vi "LVClass_WavefrontCorrector Check and Move to Absolute Position.vi"(0 "WavefrontCorrector in":refnum<class "WavefrontCorrector.lvclass">, 5 "Position":T1, 7 "Sleep after command apply (ms)":i32, 9 "Mirror preferences.Wavefront Corrector State":T2[](array[typedef]), 11 "error in (no error)":errorcluster) -> (4 "WavefrontCorrector out":refnum<class "WavefrontCorrector.lvclass">, 15 "error out":errorcluster)   [LabVIEW 2020, in "WavefrontCorrector.lvclass"]
uses:
  WavefrontCorrector.lvclass
  Wavefront Corrector states - ONE.ctl
  Wavefront Corrector Position.ctl
  Wavefront Corrector states.ctl
  WavefrontCorrector.lvclass/WavefrontCorrector.ctl
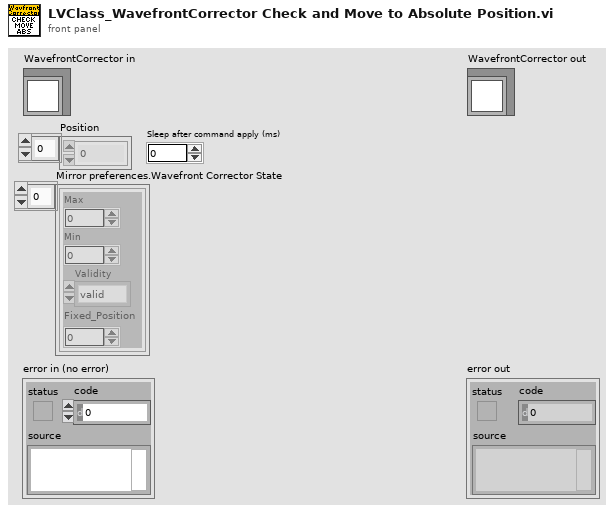
[diagram p1: front panel]
types:
  T1 = typedef "Wavefront Corrector Position.ctl" = sgl[]
  T2 = typedef "Wavefront Corrector states - ONE.ctl" = cluster{"Max":sgl, "Min":sgl, "Validity":enum16{"valid", "fixed", "invalid"}, "Fixed_Position":sgl}
  T3 = typedef "Wavefront Corrector states.ctl" = cluster{"Sleep after command apply_ms":i32, "Wavefront Corrector State":T2[], "WavefrontCorrectorOffsetState":sgl[]}
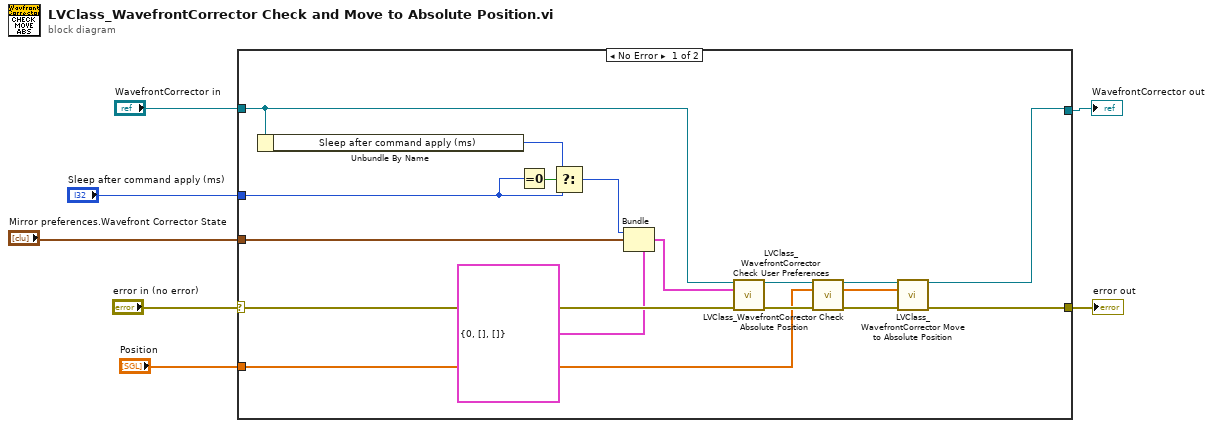
[diagram p0: block diagram]
diagram:
  n1 = case shown="No Error" "error in (no error)" {
    selector: "error in (no error)" -> [w18 w26]
    tunnel: [w22 w26] -> w4
    tunnel: [w21 w25] -> w5
    tunnel: "WavefrontCorrector in" -> [w14 w25]
    tunnel: "Sleep after command apply (ms)" -> [w13 _]
    tunnel: "Position" -> [w11 _]
    tunnel: "Mirror preferences.Wavefront Corrector State" -> [w10 _]
    frame No Error {
      n2 = Unbundle By Name(w14) -> ("Sleep after command apply (ms)"=w15:i32)
      n3 = Equal To 0?(x=w13) -> (x = 0?=w16:bool)
      n4 = Select(t=w15, s=w16, f=w13) -> (s? t:f=w12:i32)
      n5 = Bundle(cluster=T3 {"Sleep after command apply_ms"=0, "Wavefront Corrector State"=[], "WavefrontCorrectorOffsetState"=[]} ("Mirror preferences"), "Sleep after command apply_ms"=w12, "Wavefront Corrector State"=w10) -> (w8:T3)  [unwired: 1 in]
      n6 = call "LVClass_WavefrontCorrector Check User Preferences.vi"("WavefrontCorrector in"=w14, "Mirror preferences"=w8, "error in (no error)"=w18) -> ("WavefrontCorrector out"=w19:refnum<class "WavefrontCorrector.lvclass">, "error out"=w17:errorcluster)  [unwired: 11 in]
      n7 = call "LVClass_WavefrontCorrector Check Absolute Position.vi"("WavefrontCorrector in"=w19, "Absolute Positions"=w11, "error in (no error)"=w17) -> ("WavefrontCorrector out"=w24:refnum<class "WavefrontCorrector.lvclass">, "Absolute Positions OUT"=w20:T1, "error out"=w23:errorcluster)  [unwired: 10 in]
      n8 = call "LVClass_WavefrontCorrector Move to Absolute Position.vi"("WavefrontCorrector in"=w24, "Absolute Positions"=w20, "error in (no error)"=w23) -> ("WavefrontCorrector out"=w21:refnum<class "WavefrontCorrector.lvclass">, "error out"=w22:errorcluster)  [unwired: 11 in]
    }
    frame Error {
    }
  }
  "error out" <- w4
  "WavefrontCorrector out" <- w5
